vi "mqttTXdataQueueEnqueue.vi"(0 "queue":refnum<queue>, 5 "data in":u8[](array[numeric]) format="%x", 11 "error in (no error)":errorcluster) -> (15 "error out":errorcluster)   [LabVIEW 2014, in "labview-mqtt.lvlib"]
uses:
  labview-mqtt.lvlib
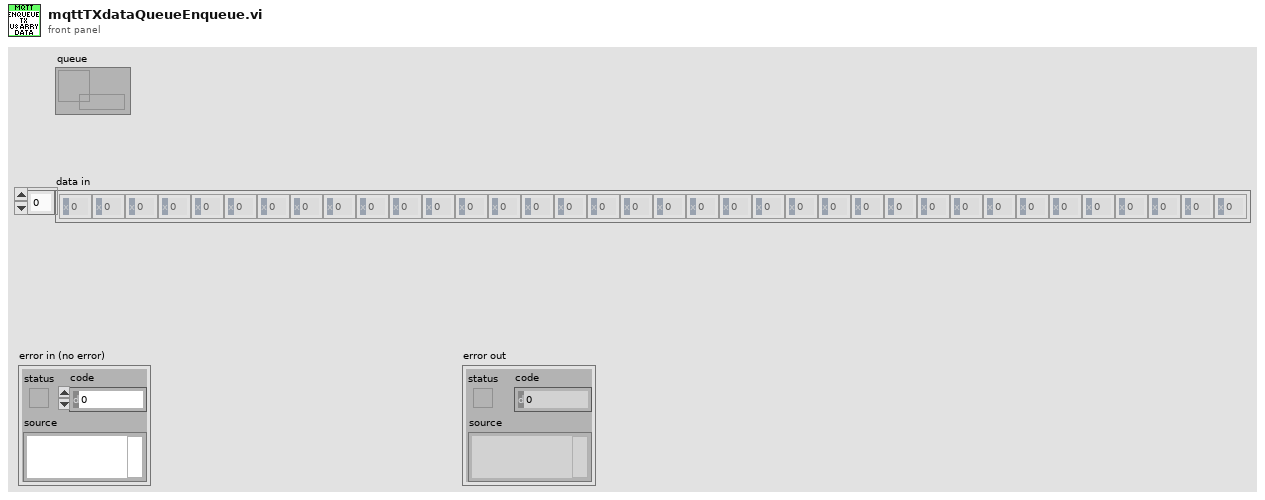
[diagram p1: front panel]
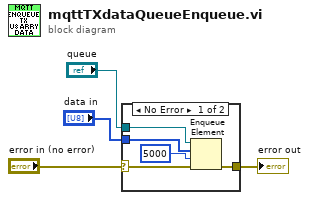
[diagram p0: block diagram]
diagram:
  n1 = case shown="No Error" "error in (no error)" {
    selector: "error in (no error)" -> [w6 w10]
    tunnel: [w5 w10] -> w3
    tunnel: "data in" -> [w7 _]
    tunnel: "queue" -> [w8 _]
    frame No Error {
      n2 = Enqueue Element(queue=w8, element=w7, timeout in ms (-1)=5000, error in (no error)=w6) -> (error out=w5:errorcluster)  [unwired: 2 out]
    }
    frame Error {
    }
  }
  "error out" <- w3
